vi "day3.vi"() -> ()   [LabVIEW 2025]
panel:
  out "subarray":string[](array[string])
  out "Array 3":string[](array[string])
  out "String 2":string
  out "sum 2":u64
  out "array w/ subset deleted 2":string[](array[string])
  out "max index(es)":i32
  out "array w/ subset deleted":string[](array[string])
  out "Array 2":i32[](array[numeric])
  out "sum":i32
  out "Array":string[](array[string])
  out "String":string
  out "string array":string[](array[string])
  in  "s":bool
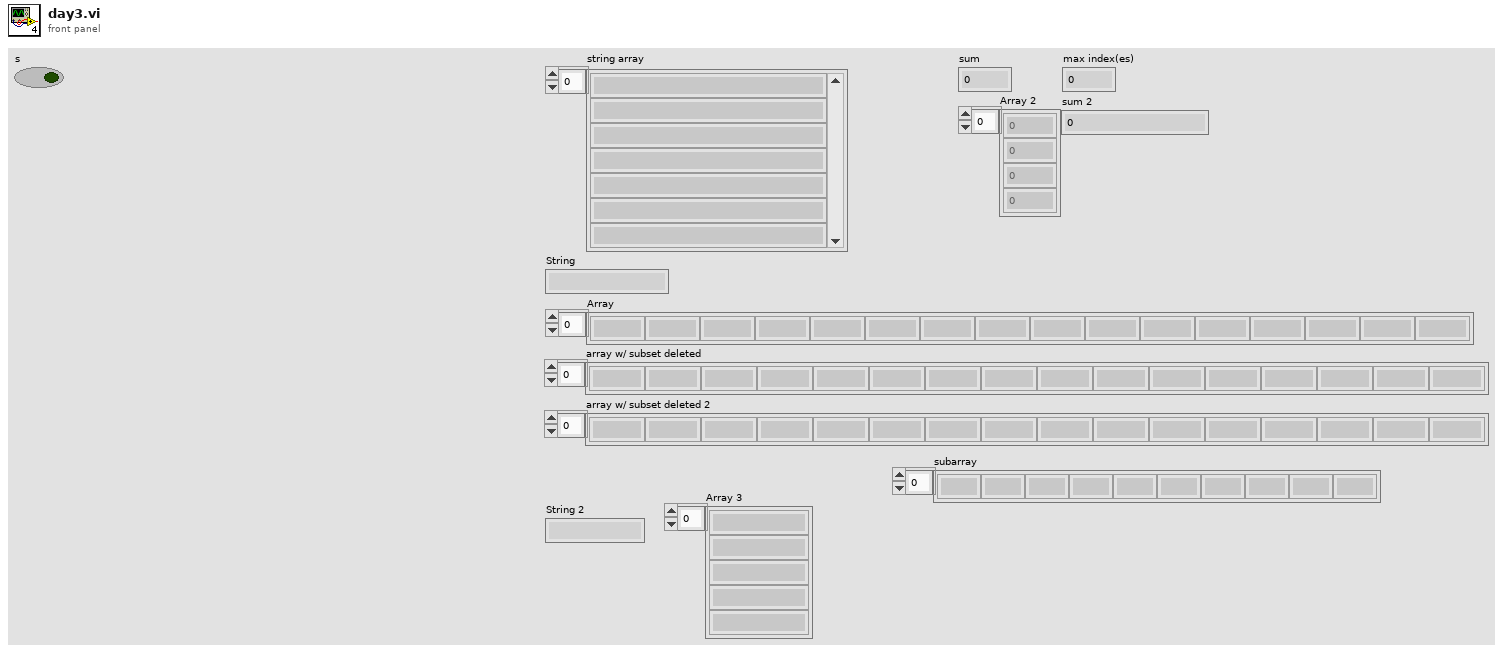
[diagram p1: front panel]
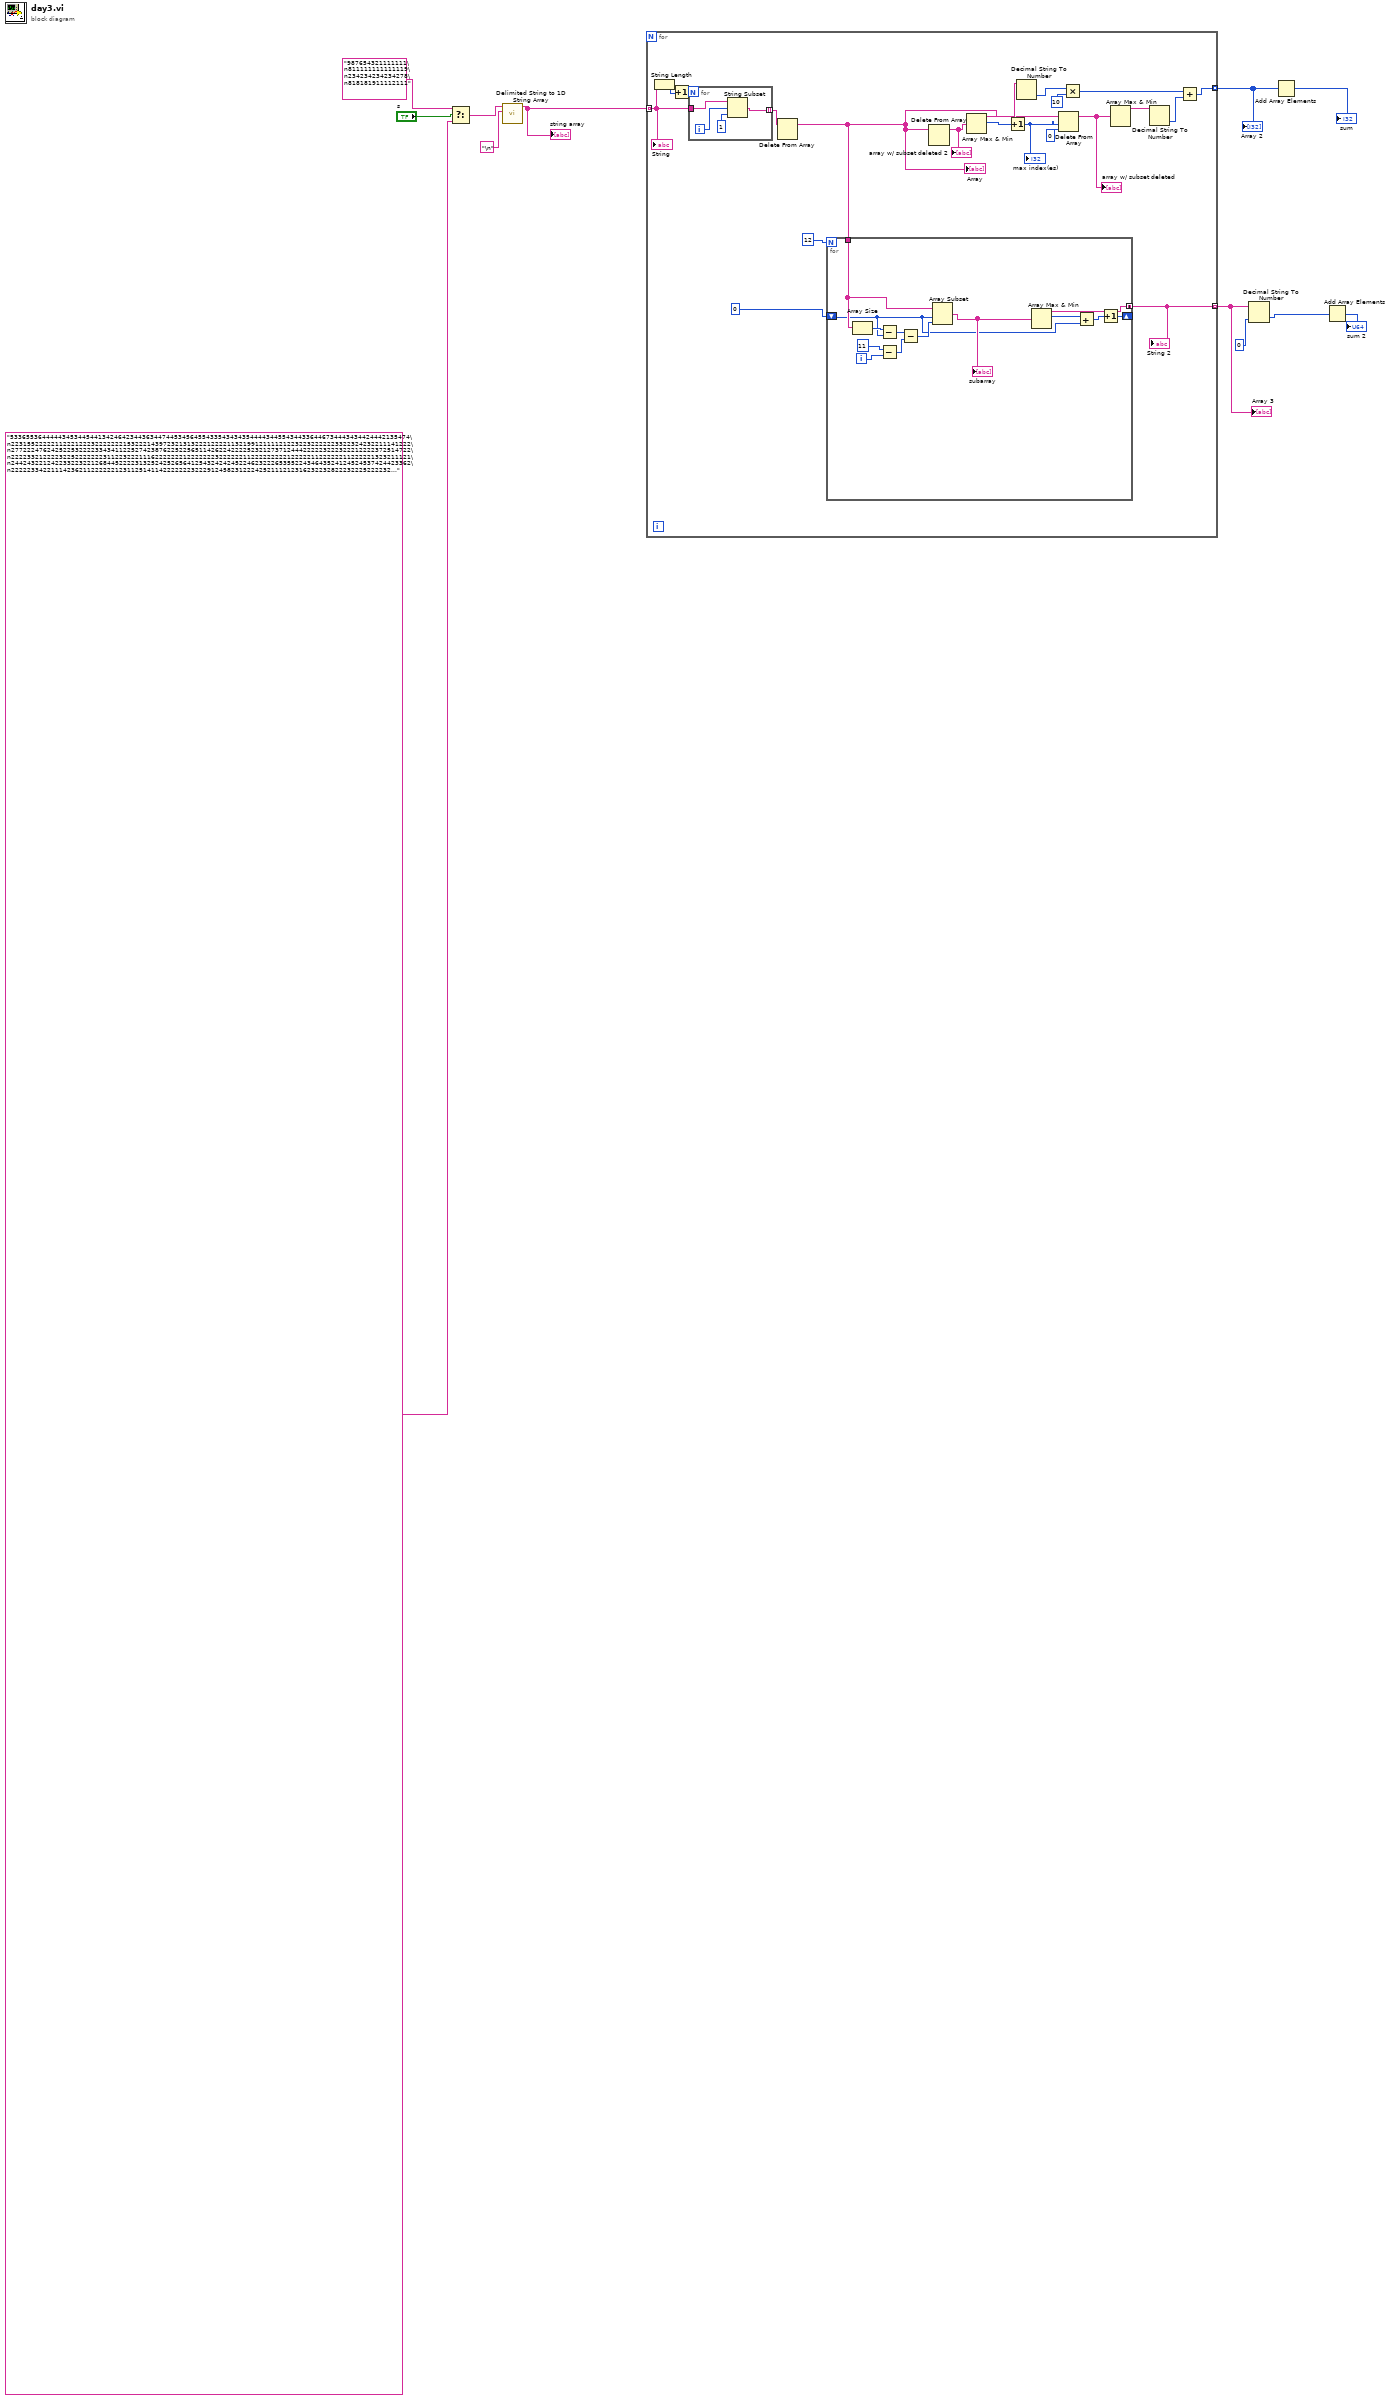
[diagram p0: block diagram]
diagram:
  n1 = Select(t="987654321111111\n811111111111119\n234234234234278\n818181911112111", s="s", f="5336553644444345344544134246423443634474453456455433543434354444344554344336446734443434424442135474\n2231552222211222122232222222153222143972321313222122221132199121111212232232222223322324232211141222\n2772224762425225322223343411225274238762252256511426224222252321273712444222223222322212222372514722\n2222332122223225222222231122322211162222222122222223222222112222222221222221122222211222221323211121\n2442432212422332232212684452222313252425265641254324242452246232226535522434643524124524537424423362\n22222334221114236211222222123112514114222222232229124582312224252111212316232232822232225222232...") -> (s? t:f=w9:string)
  n2 = call <vilib>:"Delimited String to 1D String Array.vi"("delimiter"="\n", "delimited string"=w9) -> ("string array"=w7:string[])  [unwired: 9 in]
  "string array" <- w7
  n3 = for {
    tunnel: w7 -> [w31] mode=indexing
    tunnel: [w23] -> w5 mode=indexing
    tunnel: [w13] -> w1 mode=indexing
    n4 = String Length(string=w31) -> (length=w32:i32)
    n5 = Increment(x=w32) -> (x+1=w30:i32)
    n6 = for {
      N: w30 -> [_]
      tunnel: w31 -> [w49]
      tunnel: [w48] -> w17 mode=indexing
      i -> [w46]
      n7 = String Subset(string=w49, offset (0)=w46, length (rest)=1 ("length (rest)")) -> (substring=w48:string)
    }
    n8 = Delete From Array(array=w17) -> (array with subset deleted=w14:string[])  [unwired: 2 in, 1 out]
    "Array" <- w14
    n9 = for {
      N: 12 -> [_]
      shift-right: [w33] -> _
      shift-left: 0 -> [w35]
      tunnel: w14 -> [w44]
      tunnel: [w43] -> w13 mode=concatenating
      i -> [w42]
      n10 = Array Size(array=w44) -> (size(s)=w45:i32)
      n11 = Subtract(x=w45, y=w35) -> (x-y=w40:i32)
      n12 = Subtract(x=11, y=w42) -> (x-y=w39:i32)
      n13 = Subtract(x=w40, y=w39) -> (x-y=w38:i32)
      n14 = Array Subset(array=w44, index=w35, length=w38) -> (w37:string[])
      "subarray" <- w37
      n15 = Array Max & Min(array=w37) -> (max value=w43:string, max index (indices)=w36:i32)  [unwired: 2 out]
      n16 = Add(x=w36, y=w35) -> (x+y=w34:i32)
      n17 = Increment(x=w34) -> (x+1=w33:i32)
    }
    "String 2" <- w13
    n18 = Delete From Array(array=w14) -> (array with subset deleted=w18:string[])  [unwired: 2 in, 1 out]
    "array w/ subset deleted 2" <- w18
    n19 = Array Max & Min(array=w18) -> (max value=w29:string, max index (indices)=w21:i32)  [unwired: 2 out]
    n20 = Increment(x=w21) -> (x+1=w19:i32)
    "max index(es)" <- w19
    n21 = Decimal String To Number(string=w29) -> (number=w28:i32)  [unwired: 2 in, 1 out]
    n22 = Delete From Array(array=w14, length=w19, index=0) -> (array with subset deleted=w22:string[])  [unwired: 1 out]
    "array w/ subset deleted" <- w22
    n23 = Multiply(x=w28, y=10) -> (x*y=w25:i32)
    n24 = Array Max & Min(array=w22) -> (max value=w26:string)  [unwired: 3 out]
    n25 = Decimal String To Number(string=w26) -> (number=w24:i32)  [unwired: 2 in, 1 out]
    n26 = Add(x=w25, y=w24) -> (x+y=w23:i32)
    "String" <- w31
  }
  "Array 2" <- w5
  "Array 3" <- w1
  n27 = Decimal String To Number(string=w1, default (0L)=u64 0 ("default (0 I32)")) -> (number=w4:u64[])  [unwired: 1 in, 1 out]
  n28 = Add Array Elements(numeric array=w5) -> (sum=→"sum":i32)
  n29 = Add Array Elements(numeric array=w4) -> (sum=→"sum 2":u64)
